vi "Plotter.vi"() -> ()   [LabVIEW 2009]
uses:
  <vilib>/Utility/miscctls.llb/LVPositionTypeDef.ctl
  <vilib>/Utility/tcp.llb/UDP Multicast Read-Only Open.vi
  General-Controler/Stop button.ctl
  <vilib>/Utility/file.llb/Read From Spreadsheet File (string).vi
  <userlib>/_OpenG.lib/array/array.llb/Search 1D Array (String)__ogtk.vi
  <vilib>/Utility/miscctls.llb/LVRectTypeDef.ctl
panel:
  out "Axis Name List":string[](array[string])
  out "Y Axis Default name":string
  out "All Devices Core Info":string[][](array[string])
  out "IP Addresses":string[](array[string])
  out "error out":errorcluster
  out "Position 2":T1
  out "Position":T1
  out "MY IP":string
  out "UDP Mcast Error":errorcluster
  out "Shot #":string
  in  "Tab Control 2":T2(tab)
  out "expt config file array":string[][](array[string])
  out "parameters to get":string[][](array[string])
  out "devices to get data from":string[](array[string])
  out "ScanData to receive":string[][](array[string])
  out "ShotData":string[](array[string])
  out "All shot data":string[][](array[string])
  out "TCP Ports":refnum<k5>[](array[refnum])
  out "Array":errorcluster[](array[cluster])
  in  "Tab Control":enum32{"Main", "ShotData", "setup"}(tab)
  out "xy graph":cluster{dbl[], dbl[]}(graph)={[1.0, 1.0, 1.0, 1.0, 1.0, 1.0, 1.0], [-1.0, -1.0, -1.0, -1.0, -1.0, -1.0, -1.0]}
  in  "Y Axis":u16(ring) items=["Cam1 exposure", "Cam1 trigger", "Cam1 gain", "Cam1Analysis centroidx"]
  in  "X Axis":u16(ring)=1 items=["Cam1 exposure", "Cam1 trigger", "Cam1 gain", "Cam1Analysis centroidx"]
  in  "OK Button":bool
  out "Energy transmission 2":cluster{"y vector":dbl[], "avg optspec":dbl[]}[](graph)
  in  "Fixed Interval":bool
  in  "Interval":dbl format="%.3p"
  in  "Auto Interval":bool
  in  "Error Bar Type":T3(ring)
  in  "Experiment":u16(ring) items=["Cam1only.txt", "Test Startup config.txt", "TREX-Standard.txt"]
  out "Current State":string
  out "Mcast Data":string
  out "Devices Data Timed out":string[](array[string])
  in  "Left":i16=25
  in  "Top":i16=75
  out "x axis name":string
  in  "TCP Open timeout ms":i32=300
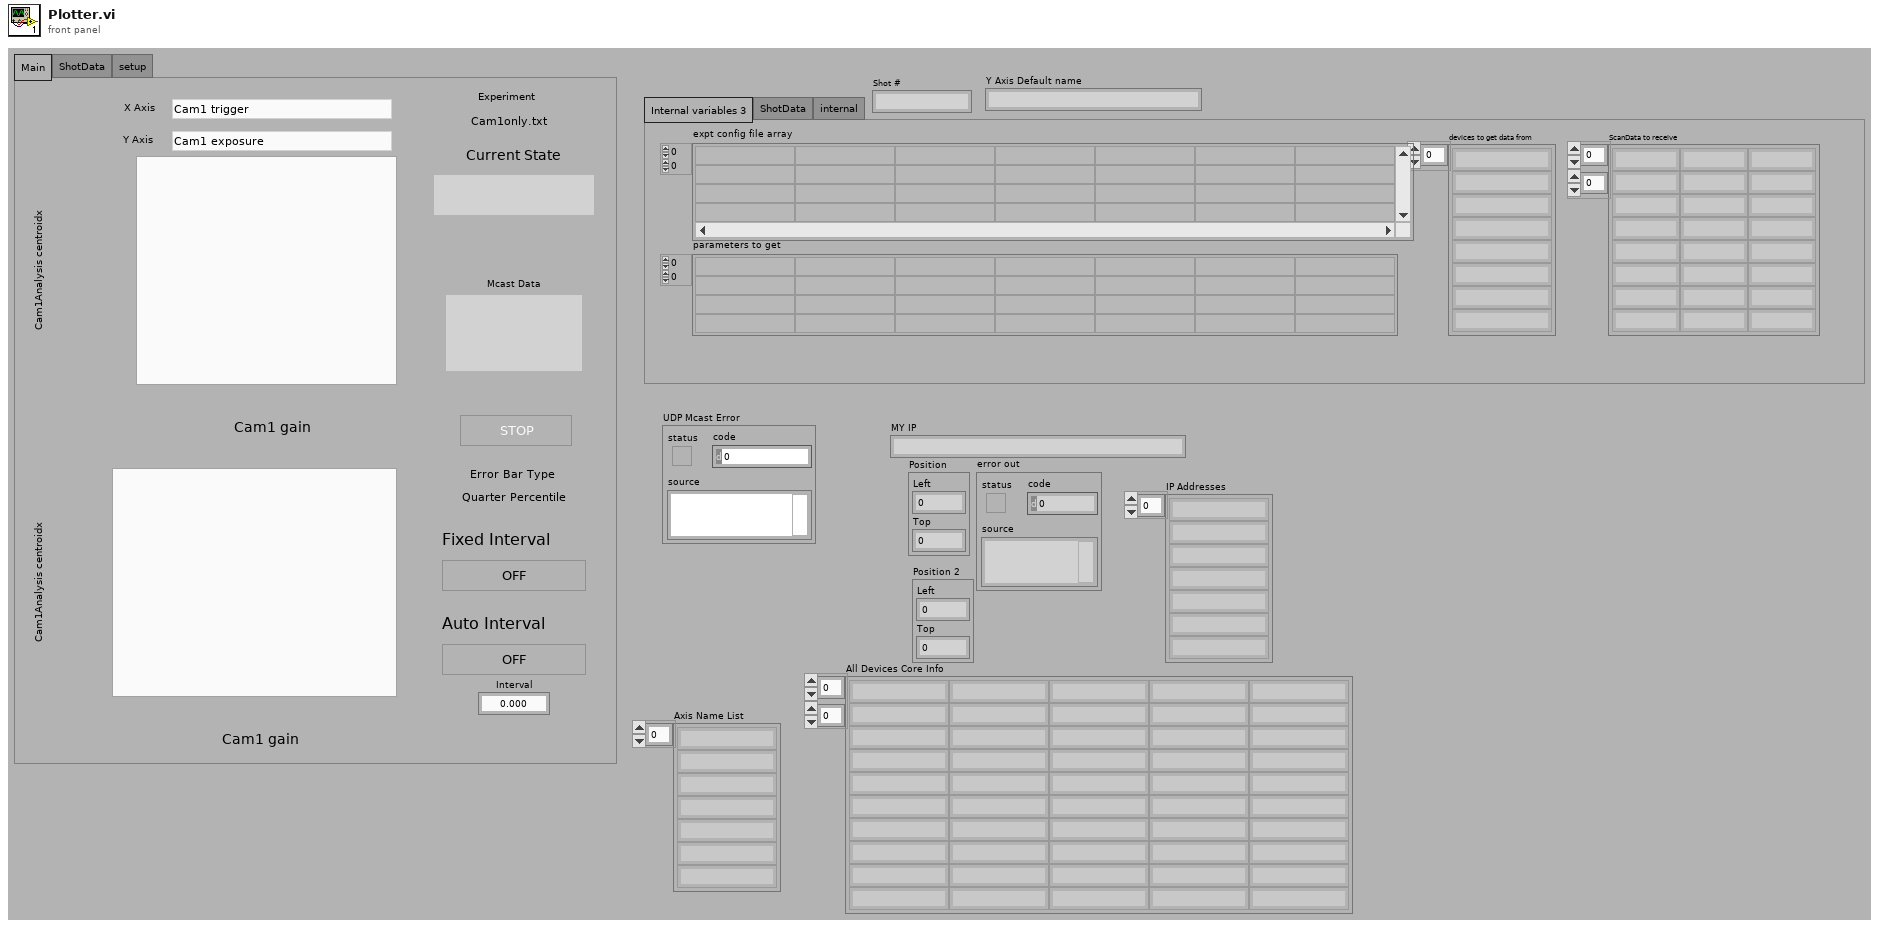
[diagram p1: front panel]
types:
  T1 = typedef "LVPositionTypeDef.ctl" = cluster{"Left":i32, "Top":i32}
  T2 = enum32{"Internal variables 3", "ShotData", "internal"}
  T3 = enum16{"Quarter Percentile", "Standard Deviation"}
  T4 = typedef "Stop button.ctl" = bool
  T5 = enum32{"invalid app kind", "Development System", "Run Time System", "Student Edition", "Embedded LabVIEW", "Evaluation", "Custom"}
  T6 = enum32{"Invalid", "Standard", "Closed", "Hidden", "Minimized", "Maximized"}
  T7 = typedef "LVRectTypeDef.ctl" = cluster{"Left":i16, "Top":i16, "Right":i16, "Bottom":i16}
  T8 = cluster{"Core":cluster{"Current VI Reference":refnum<vi>, "Close Panel on Exit?":bool}, "Variable selector":u16, "variable parameters":string[], "list of variables":string[], "UDP Command to send":string, "Device List":string[], "Config path":path, "Devices Selector":u16, "Device Config file array":string[][], "All Devices Core Info":string[][], "Location Filter":u16, "Filtered Device List":string[], "Class Filter":u16, "Command to Send":string, "Devices Path":path, "UDP ID":refnum<k16>, "parameter vals scanned":dbl[], "List Commands Not Executed":string[], "Expected slow response":string, "MCast Address":string, "MCast Local Port":u16, "MCast Remote Port":u16, "UDP timeout ms":i32, "Scan Number":i32, "Shot Number":i32, "Scan Data Titles":string[], "Scan Data Array":dbl[], "Expt Config Files":string[], "Experiment name":string, "UDP fast port":u16, "name":string, "ScanData to receive":string[][], "UDP Listen Ports":u16[], "Device Names for scan data":string[], "ShotData":string[], "Scans Path":path, "Device xxx Path":path, "numeric?":bool, "Last Slow response":string, "Mcast command":string, "Device Status Array":bool[], "expt config file array":string[][], "Shot Data plotter":string[][], "Data titles from config array":string[]}
  T9 = typedef "LVPointTypeDef.ctl" = cluster{"Horizontal":i16, "Vertical":i16}
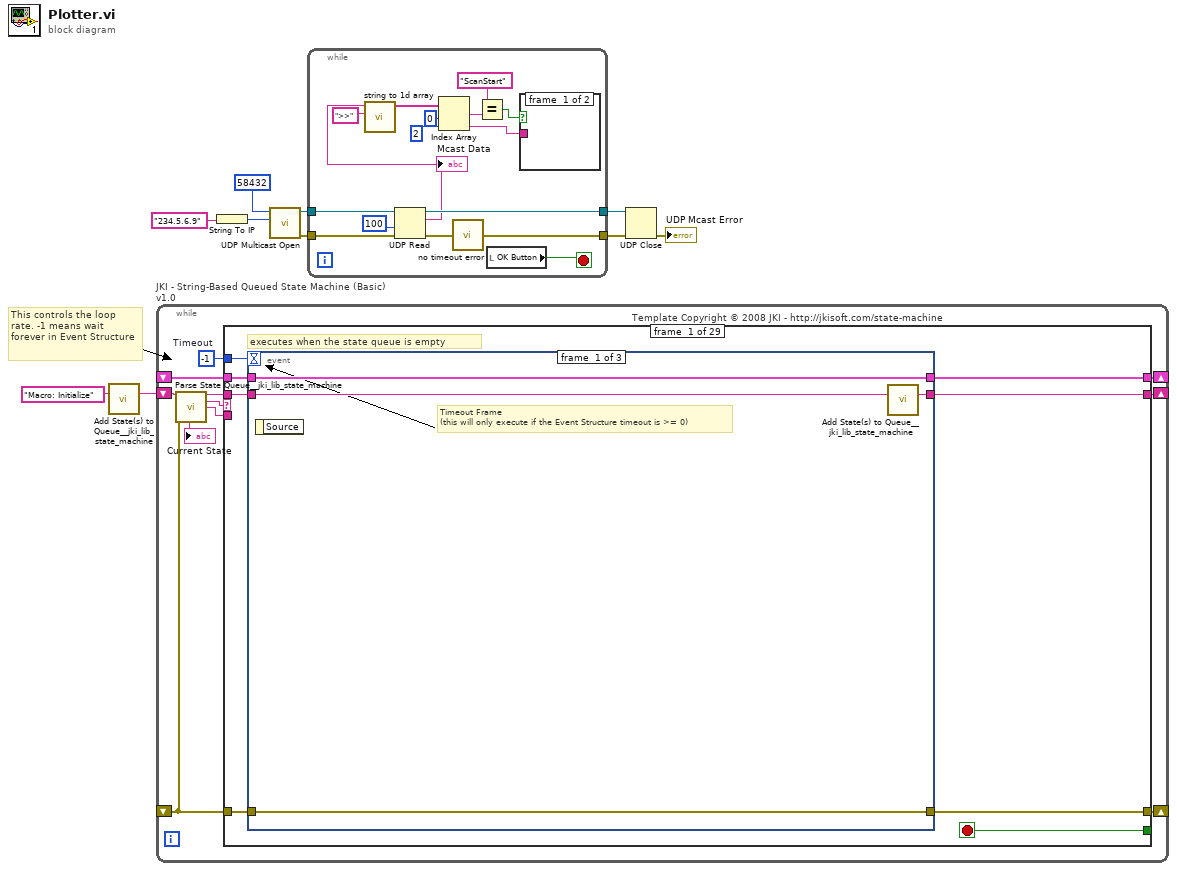
[diagram p0: block diagram]
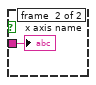
[diagram p2: hidden frame]
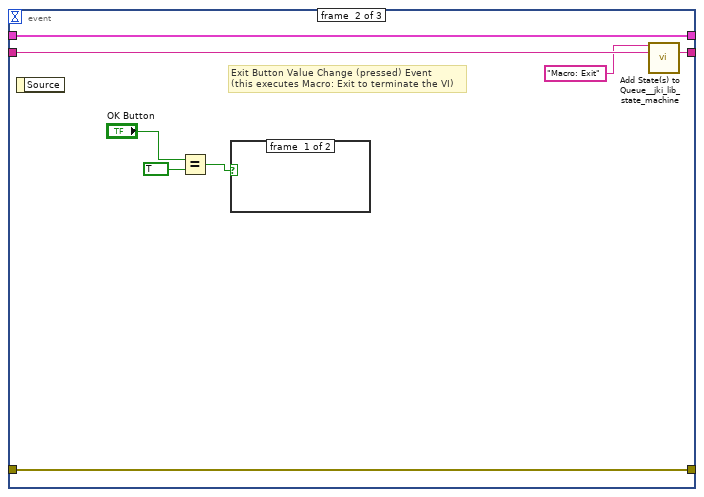
[diagram p3: hidden frame]
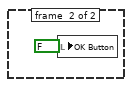
[diagram p4: hidden frame]
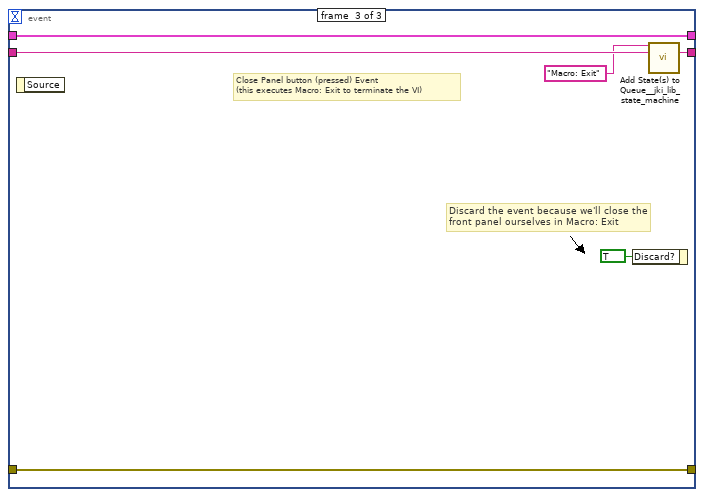
[diagram p5: hidden frame]
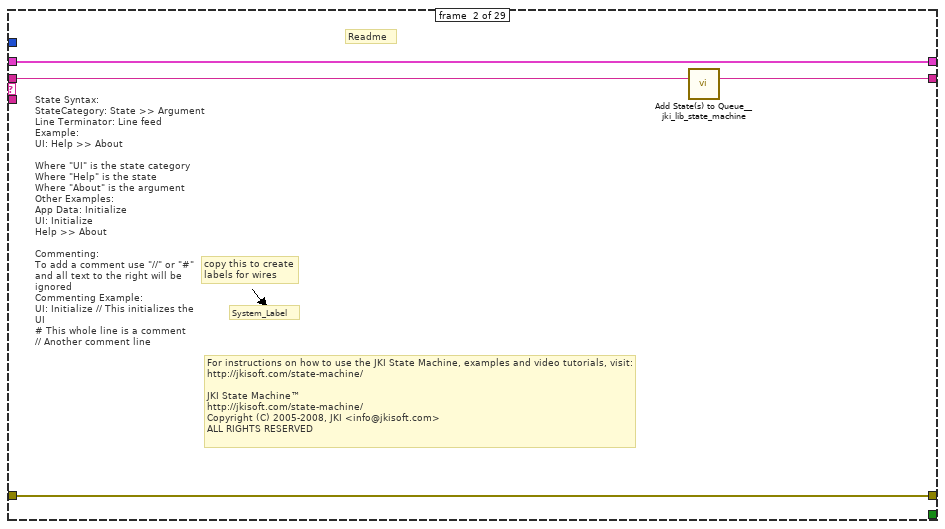
[diagram p6: hidden frame]
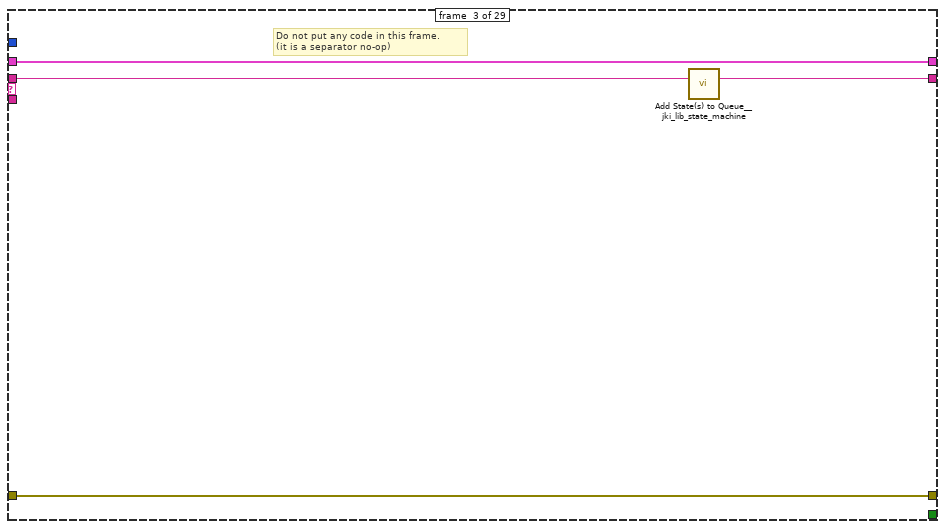
[diagram p7: hidden frame]
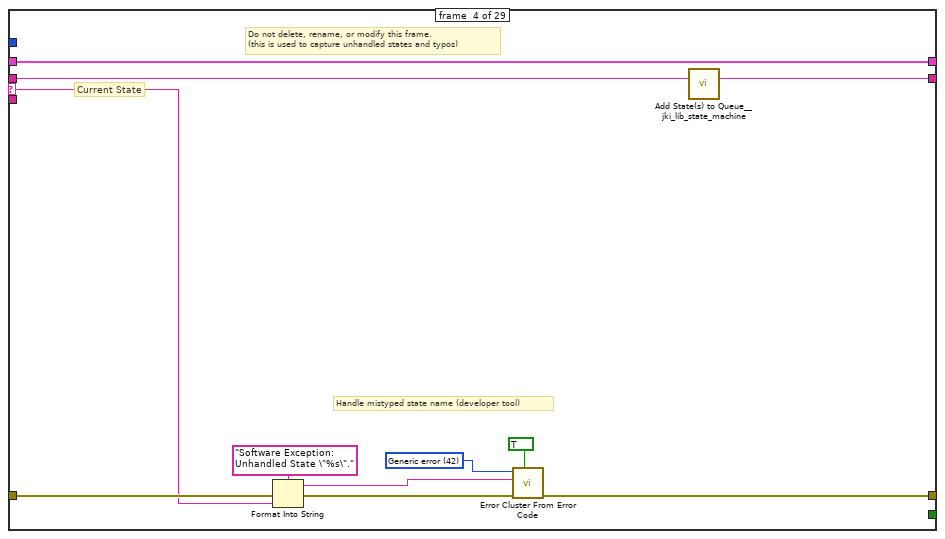
[diagram p8: hidden frame]
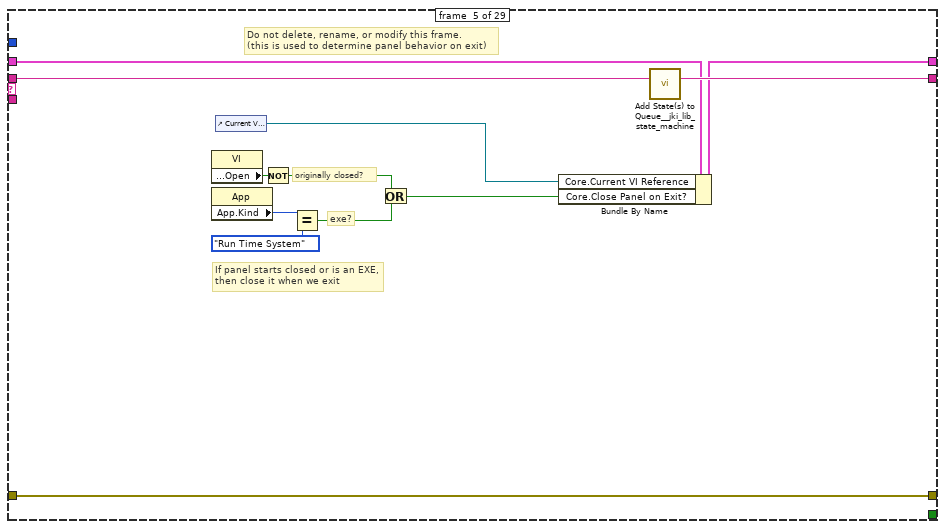
[diagram p9: hidden frame]
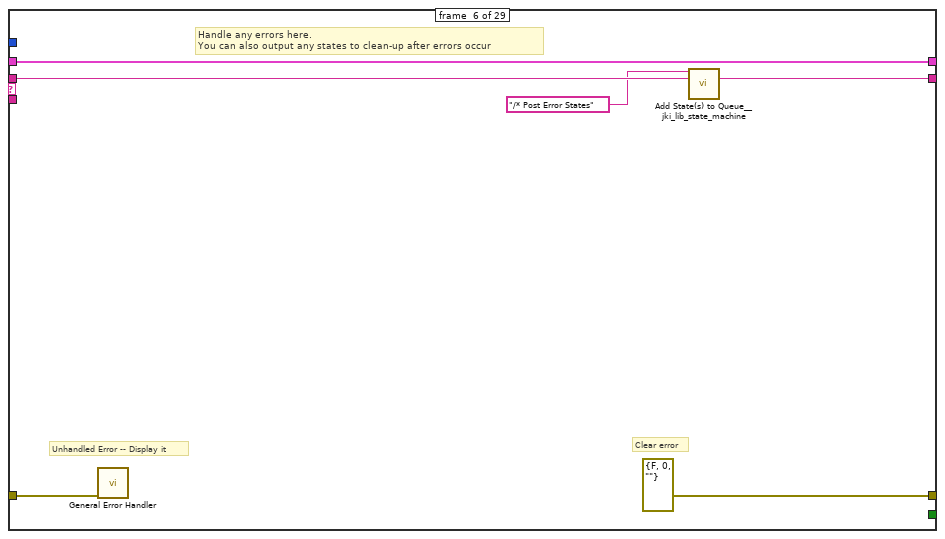
[diagram p10: hidden frame]
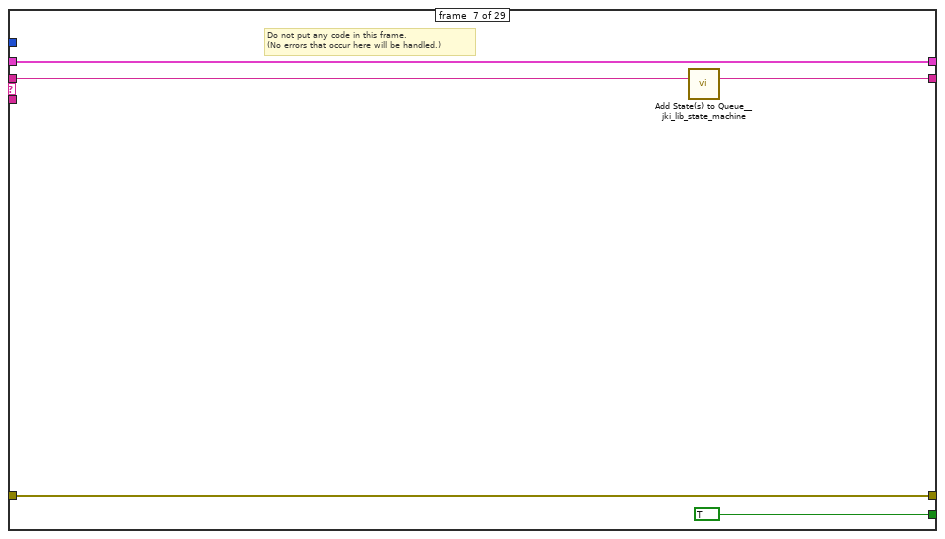
[diagram p11: hidden frame]
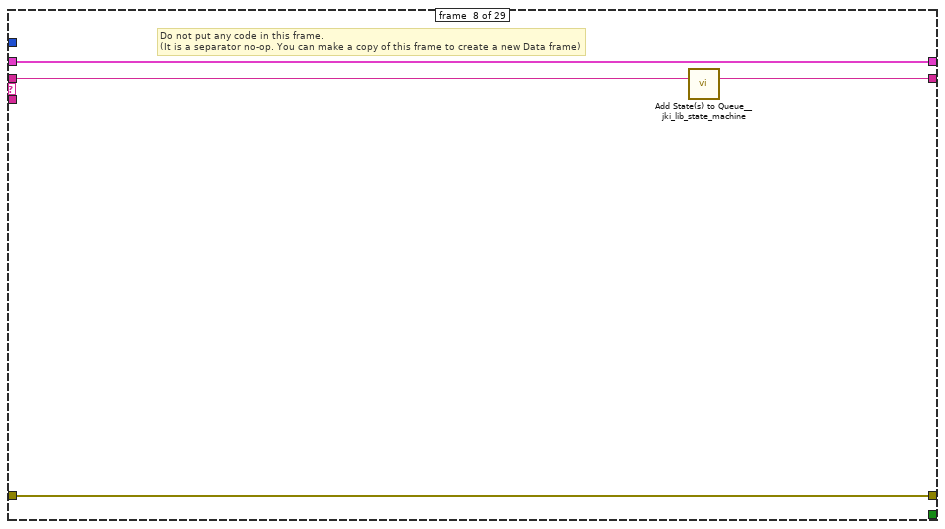
[diagram p12: hidden frame]
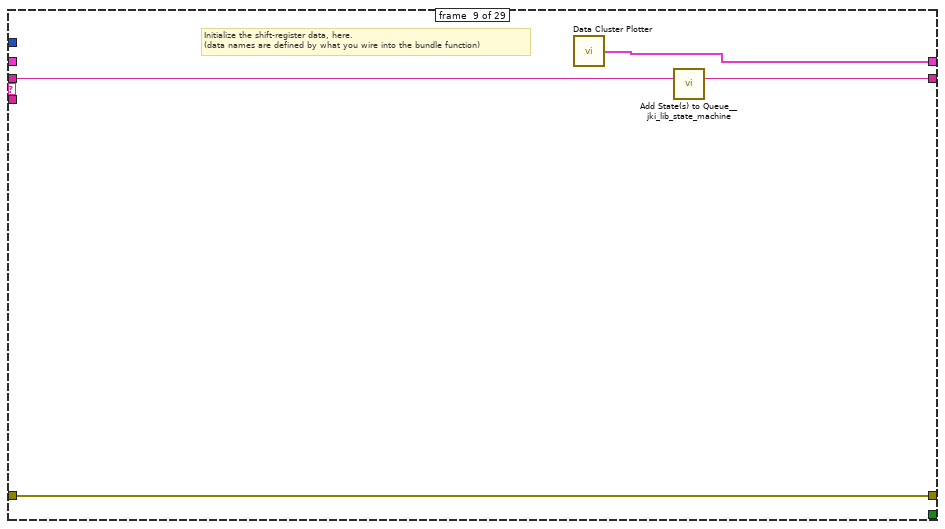
[diagram p13: hidden frame]
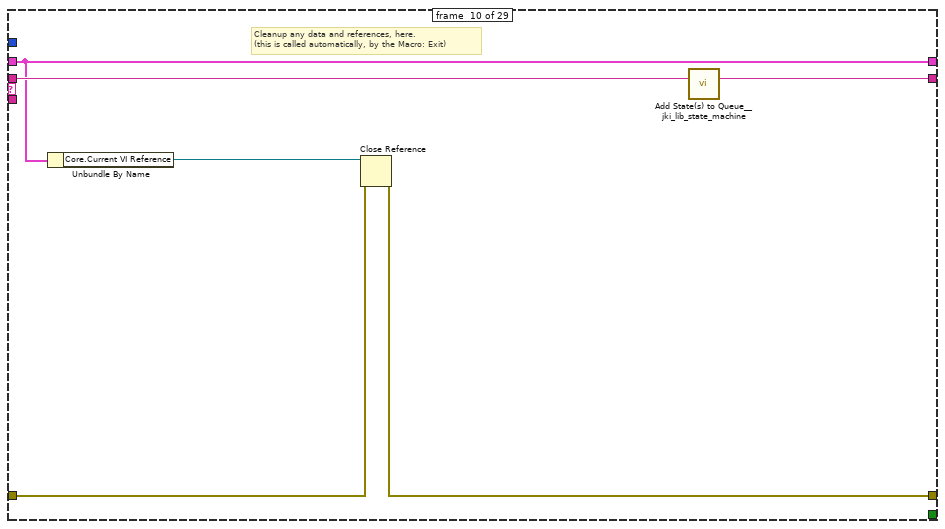
[diagram p14: hidden frame]
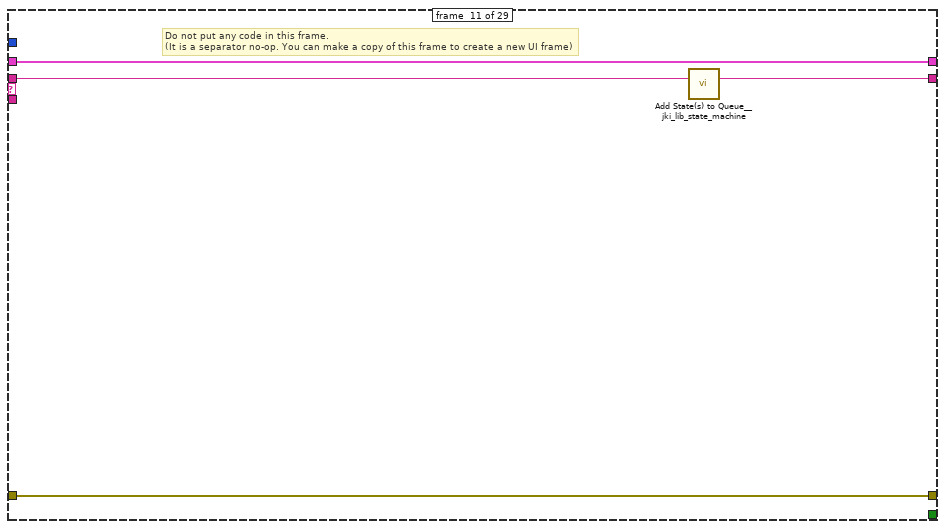
[diagram p15: hidden frame]
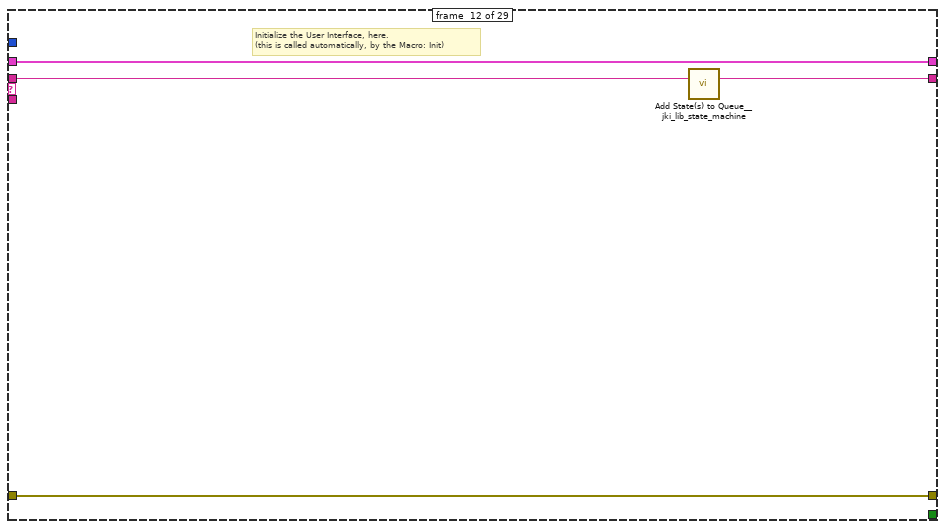
[diagram p16: hidden frame]
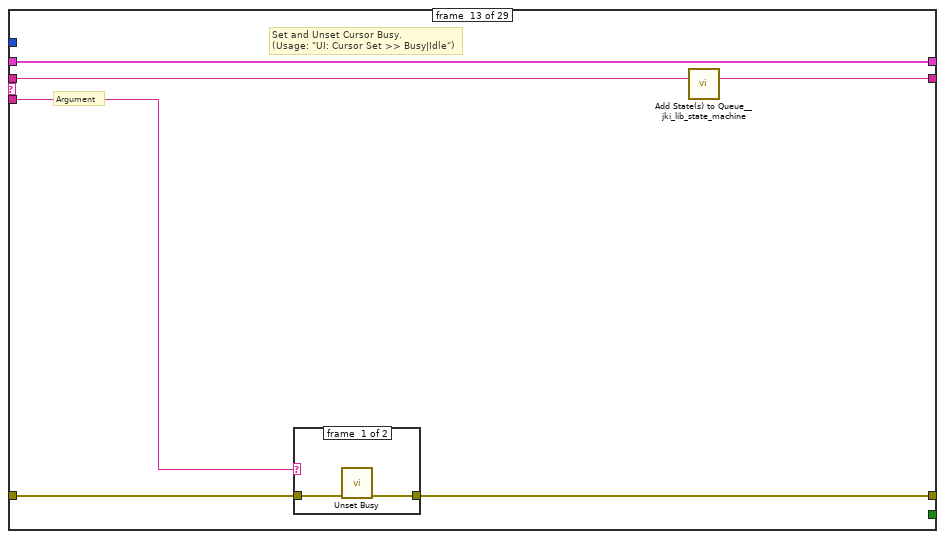
[diagram p17: hidden frame]
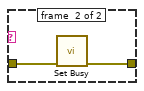
[diagram p18: hidden frame]
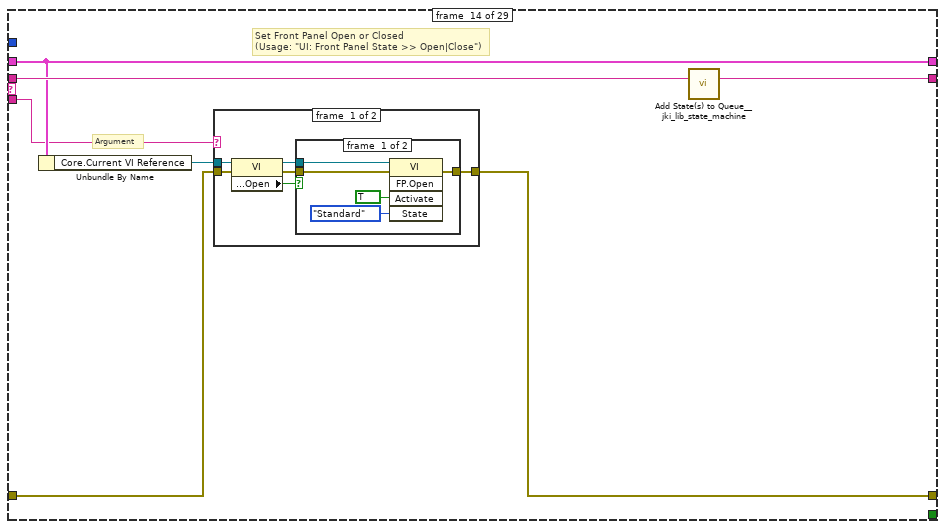
[diagram p19: hidden frame]
diagram:
  # "This controls the loop rate. -1 means wait forever in Event Structure"
  n1 = call <vilib>:"Add State(s) to Queue__jki_lib_state_machine.vi"("State(s) in (\"\")"="Macro: Initialize") -> ("States Out"=w10:string)  [unwired: 14 in]
  n2 = while "JKI - String-Based Queued State Machine (Basic) v1.0" {
    shift-right: [w14] -> _
    shift-left: _ -> [w13]
    shift-right: [w17] -> _
    shift-left: _ -> [w11]
    shift-right: [w16] -> _
    shift-left: w10 -> [w18]
    stop <- w15 stop-if-true
    w12 = -1  # Timeout
    # "Template Copyright © 2008 JKI - http://jkisoft.com/state-machine"
    n3 = call <vilib>:"Parse State Queue__jki_lib_state_machine.vi"("State Queue"=w18, "Error In (no error)"=w11) -> ("Remaining States"=w20:string, "Current State"=w21:string, "Arguments"=w19:string)  [unwired: 11 in]
    "Current State" <- w21
    n4 = case shown="\"Get List of Axis Names\"" w21 {
      selector: w21 -> [_ _ _ w56 _ _ _ _ _ _ _ _ _ _ _ _ _ _ _ _ _ _ _ _ _ _ _ _ _]
      tunnel: w20 -> [w28 w51 w55 w60 w78 w84 w89 w93 w97 w103 w107 w111 w117 w128 w154 w159 w169 w173 w179 w188 w196 w218 w232 w255 w283 w291 w307 w326 w380]
      tunnel: w19 -> [_ _ _ _ _ _ _ _ _ _ _ _ w112 w122 _ _ _ _ _ _ _ _ _ _ _ _ _ _ _]
      tunnel: w13 -> [w26 w48 w52 w58 w69 w81 w87 w90 _ w98 w104 w109 w115 w124 w151 w155 w167 w170 w176 w183 w194 w211 w223 w244 w280 w284 w295 w322 w377]
      tunnel: [w25 w49 w53 w62 w75 errorcluster {"status"=FALSE, "code"=0, "source"=""} ("error out") w86 w91 w95 w99 w105 w108 w113 w125 w152 w157 w160 w171 w177 w180 w191 w199 w230 w253 w281 w289 w293 w324 w378] -> w17
      tunnel: w11 -> [w24 w49 w53 w61 w75 w80 w86 w91 w95 w100 w105 w108 w114 w126 w152 w157 w160 w171 w177 w181 w191 w200 w230 w253 w281 w289 w293 w324 w378]
      tunnel: [w27 w50 w54 w59 w77 w83 w88 w92 w96 w102 w106 w110 w116 w127 w153 w158 w168 w172 w178 w187 w195 w217 w231 w254 w282 w290 w306 w325 w379] -> w16
      tunnel: [_ _ _ _ _ _ TRUE _ _ _ _ _ _ _ _ _ _ _ _ _ _ _ _ _ _ _ _ _ _] -> w15
      tunnel: [w23 w48 w52 w58 w76 w81 w87 w90 w94 w98 w104 w109 w115 w124 w151 w155 w167 w170 w176 w182 w193 w210 w222 w244 w280 w285 w295 w322 w377] -> w14
      tunnel: w12 -> [w22 _ _ _ _ _ _ _ _ _ _ _ _ _ _ _ _ _ _ _ _ _ _ _ _ _ _ _ _]
      frame #0 {
        # "executes when the state queue is empty"
        n5 = event shown="[1] \"OK Button\": Value Change" {
          selector: _ -> [_ _ _]
          dyn-events: _ -> [_ _ _]
          timeout: w22 -> [_ _ _]
          tunnel: w28 -> [w32 w40 w47]
          tunnel: [w31 w39 w46] -> w27
          tunnel: w26 -> [w29 w37 w44]
          tunnel: [w30 w38 w45] -> w25
          tunnel: w24 -> [w30 w38 w45]
          tunnel: [w29 w37 w44] -> w23
          event #0 {
            # "Timeout Frame\n(this will only execute if the Event Structure timeout is >= 0)"
            n6 = event-data() -> ()  [unwired: 1 in, 1 out]
            n7 = call <vilib>:"Add State(s) to Queue__jki_lib_state_machine.vi"("State(s) in (\"\")"=w32) -> ("States Out"=w31:string)  [unwired: 14 in]
          }
          event #1 {
            # "Exit Button Value Change (pressed) Event\n(this executes Macro: Exit to terminate the VI)"
            n8 = event-data() -> ()  [unwired: 1 in, 1 out]
            n9 = Equal?(x="OK Button", y=T4 TRUE) -> (x = y?=w33:T4)
            n10 = case shown="True" w33 {
              frame #0 {
              }
              frame #1 {
                n11 = local write "OK Button"(T4 FALSE ("STOP")) -> ()
              }
            }
            n12 = call <vilib>:"Add State(s) to Queue__jki_lib_state_machine.vi"("State(s) in Front (\"\")"="Macro: Exit", "State(s) in (\"\")"=w40) -> ("States Out"=w39:string)  [unwired: 13 in]
          }
          event #2 {
            # "Discard the event because we'll close the front panel ourselves in Macro: Exit"
            # "Close Panel button (pressed) Event\n(this executes Macro: Exit to terminate the VI)"
            n13 = event-data() -> ()  [unwired: 1 in, 1 out]
            n14 = event-data("Discard?"=TRUE) -> ()  [unwired: 1 in, 1 out]
            n15 = call <vilib>:"Add State(s) to Queue__jki_lib_state_machine.vi"("State(s) in Front (\"\")"="Macro: Exit", "State(s) in (\"\")"=w47) -> ("States Out"=w46:string)  [unwired: 13 in]
          }
        }
      }
      frame #1 {
        # "For instructions on how to use the JKI State Machine, examples and video tutorials, visit:\nhttp://jkisoft.com/state-machine/\n\nJKI State Machine™\nhttp://jkisoft.com/state-machine/\nCopyright (C) 2005-2008, JKI <info@jkisoft.com>\nALL RIGHTS RESERVED"
        # "copy this to create labels for wires"
        # "System_Label"
        # "State Syntax:\nStateCategory: State >> Argument\nLine Terminator: Line feed\nExample:\nUI: Help >> About\n\nWhere \"UI\" is the state category\nWhere \"Help\" is the state\nWhere \"About\" is the argument\nOther Examples:\nApp Data: Initialize\nUI: Initialize\nHelp >> About\n\nCommenting:\nTo add a comment use \"//\" or \"#\" and all text to the right will be ignored\nCommenting Example:\nUI: Initialize // This initializes the UI\n# This whole line is a comment\n// Another comment line"
        # "Readme"
        n16 = call <vilib>:"Add State(s) to Queue__jki_lib_state_machine.vi"("State(s) in (\"\")"=w51) -> ("States Out"=w50:string)  [unwired: 14 in]
      }
      frame #2 {
        # "Do not put any code in this frame.\n(it is a separator no-op)"
        n17 = call <vilib>:"Add State(s) to Queue__jki_lib_state_machine.vi"("State(s) in (\"\")"=w55) -> ("States Out"=w54:string)  [unwired: 14 in]
      }
      frame #3 {
        w65 = 42 items=["No error", "Argument error", "Memory is full", "Out of zone", "End of file", "File already open", "Generic file I/O error", "File not found", "File permission error", "Disk is full", "Duplicate path", "Too many files open", "System feature not enabled", "Resource file not found", "Cannot add resource", "Resource not found", "Image not found", "Image memory error", "Pen does not exist", "Config type invalid", "Config token not found", "Config parse error", "Config memory error", "Bad external code format", "Bad external code offset", "External code not present", "Null window", "Destroy window error", "Null menu", "Print aborted", "Bad print record", "Print driver error", "Windows error during printing", "Memory error during printing", "Print dialog error", "Generic print error", "Invalid device refnum", "Device not found", "Device parameter error", "Device unit error", "Cannot open device", "Device call aborted", "Generic error", "Cancelled by user", "Object ID too low", "Object ID too high", "Object not in heap", "Unknown heap", "Unknown object (invalid DefProc)", "Unknown object (DefProc not in table)", "Message out of range", "Invalid (null) method", "Unknown message", "Manager call not supported", "Bad address", "Network operation in progress", "Network operation timed out", "Connection is busy", "Network attribute not supported", "Network error", "Address in use", "System out of memory", "Connection aborted", "Connection refused", "Not connected", "Already connected", "Connection closed", "Initialization error (interapplication manager)", "Bad occurrence", "Wait on unbound occurrence handler", "Occurrence queue overflow", "Datalog type conflict", "Unused", "Unrecognized type (interapplication manager)", "Memory corrupt", "Failed to make temporary DLL", "Old CIN version", "Drag socket not found", "Failed to load drop-object", "Failed to register OLE object", "Failed to release OLE object", "Format specifier type mismatch", "Unknown format specifier", "Too few format specifiers", "Too many format specifiers", "Scan failed", "Newer CIN version", "Error converting to variant", "Runtime menu error", "Password tampered", "Variant attribute not found", "Incompatible variant data type", "Event data is not available", "Event Store is not present", "Occurrence is not found", "Event Queue is not created", "Event info is not available", "Refnum passed is NULL", "Error retrieving Class GUID", "Error retrieving CoClass GUID", "Error retrieving TypeLib GUID.", "Bad built application magic bytes.", "Specific driver is different from the specific driver associated with the Logical Name.", "There is no session opened to the class driver.", "Max Error", "MAX - Error with config objects", "MAX - Error loading configuration", "MAX - Group not supported"]
        # "Current State"
        # "Do not delete, rename, or modify this frame.\n(this is used to capture unhandled states and typos)"
        # "Handle mistyped state name (developer tool)"
        n18 = Format Into String(format string="Software Exception: Unhandled State \"%s\"." ("message"), error in=w61, w56) -> (resulting string=w64:string, error out=w63:errorcluster)  [unwired: 1 in]
        n19 = call <vilib>:"Error Cluster From Error Code.vi"("show call chain? (False)"=TRUE, "error in (no error)"=w63, "error message (\"\")"=w64, "error code (0)"=w65) -> ("error out"=w62:errorcluster)  [unwired: 5 in]
        n20 = call <vilib>:"Add State(s) to Queue__jki_lib_state_machine.vi"("State(s) in (\"\")"=w60) -> ("States Out"=w59:string)  [unwired: 14 in]
      }
      frame #4 {
        # "Do not delete, rename, or modify this frame.\n(this is used to determine panel behavior on exit)"
        # "originally closed?"
        # "exe?"
        # "If panel starts closed or is an EXE, then close it when we exit"
        n21 = property class="VI"() -> ("Front Panel.Open"=w74:bool)  [unwired: 2 in, 2 out]
        n22 = property class="App"() -> ("App.Kind"=w73:T5)  [unwired: 2 in, 2 out]
        n23 = control-ref of="Current VI Reference"() -> (w67:refnum<vi>)
        n24 = Not(x=w74) -> (.not. x?=w71:bool)
        n25 = Equal?(x=w73, y=T5."Run Time System" ("Application:Kind")) -> (x = y?=w70:bool)
        n26 = Or(x=w71, y=w70) -> (x .or. y?=w68:bool)
        n27 = Bundle By Name(cluster=w69, "Core.Current VI Reference"=w67, "Core.Close Panel on Exit?"=w68) -> (w76:T8)
        n28 = call <vilib>:"Add State(s) to Queue__jki_lib_state_machine.vi"("State(s) in (\"\")"=w78) -> ("States Out"=w77:string)  [unwired: 14 in]
      }
      frame #5 {
        # "Unhandled Error -- Display it"
        # "Handle any errors here.\nYou can also output any states to clean-up after errors occur"
        # "Clear error"
        n29 = call <vilib>:"General Error Handler.vi"("error in (no error)"=w80) -> ()  [unwired: 10 in, 5 out]
        n30 = call <vilib>:"Add State(s) to Queue__jki_lib_state_machine.vi"("State(s) in Front (\"\")"="/* Post Error States", "State(s) in (\"\")"=w84) -> ("States Out"=w83:string)  [unwired: 13 in]
      }
      frame #6 {
        # "Do not put any code in this frame.\n(No errors that occur here will be handled.)"
        n31 = call <vilib>:"Add State(s) to Queue__jki_lib_state_machine.vi"("State(s) in (\"\")"=w89) -> ("States Out"=w88:string)  [unwired: 14 in]
      }
      frame #7 {
        # "Do not put any code in this frame.\n(It is a separator no-op. You can make a copy of this frame to create a new Data frame)"
        n32 = call <vilib>:"Add State(s) to Queue__jki_lib_state_machine.vi"("State(s) in (\"\")"=w93) -> ("States Out"=w92:string)  [unwired: 14 in]
      }
      frame #8 {
        # "Initialize the shift-register data, here.\n(data names are defined by what you wire into the bundle function)"
        n33 = call "Data Cluster Plotter.vi"() -> ("output cluster"=w94:T8)
        n34 = call <vilib>:"Add State(s) to Queue__jki_lib_state_machine.vi"("State(s) in (\"\")"=w97) -> ("States Out"=w96:string)  [unwired: 14 in]
      }
      frame #9 {
        # "Cleanup any data and references, here.\n(this is called automatically, by the Macro: Exit)"
        n35 = Unbundle By Name(w98) -> ("Core.Current VI Reference"=w101:refnum<vi>)
        n36 = Close Reference(reference=w101, error in (no error)=w100) -> (error out=w99:errorcluster)
        n37 = call <vilib>:"Add State(s) to Queue__jki_lib_state_machine.vi"("State(s) in (\"\")"=w103) -> ("States Out"=w102:string)  [unwired: 14 in]
      }
      frame #10 {
        # "Do not put any code in this frame.\n(It is a separator no-op. You can make a copy of this frame to create a new UI frame)"
        n38 = call <vilib>:"Add State(s) to Queue__jki_lib_state_machine.vi"("State(s) in (\"\")"=w107) -> ("States Out"=w106:string)  [unwired: 14 in]
      }
      frame #11 {
        # "Initialize the User Interface, here.\n(this is called automatically, by the Macro: Init)"
        n39 = call <vilib>:"Add State(s) to Queue__jki_lib_state_machine.vi"("State(s) in (\"\")"=w111) -> ("States Out"=w110:string)  [unwired: 14 in]
      }
      frame #12 {
        # "Argument"
        # "Set and Unset Cursor Busy.\n(Usage: \"UI: Cursor Set >> Busy|Idle\")"
        n40 = case shown="\"Idle\", Default" w112 {
          tunnel: w114 -> [w119 w121]
          tunnel: [w118 w120] -> w113
          frame #0 {
            n41 = call <vilib>:"Unset Busy.vi"("error in (no error)"=w119) -> ("error out"=w118:errorcluster)  [unwired: 10 in]
          }
          frame #1 {
            n42 = call <vilib>:"Set Busy.vi"("error in (no error)"=w121) -> ("error out"=w120:errorcluster)  [unwired: 9 in, 1 out]
          }
        }
        n43 = call <vilib>:"Add State(s) to Queue__jki_lib_state_machine.vi"("State(s) in (\"\")"=w117) -> ("States Out"=w116:string)  [unwired: 14 in]
      }
      frame #13 {
        # "Argument"
        # "Set Front Panel Open or Closed\n(Usage: \"UI: Front Panel State >> Open|Close\")"
        n44 = Unbundle By Name(w124) -> ("Core.Current VI Reference"=w123:refnum<vi>)
        n45 = case shown="\"Open\", Default" w122 {
          tunnel: w126 -> [w132 w145]
          tunnel: [w134 w146] -> w125
          tunnel: w123 -> [w133 w143]
          frame #0 {
            n46 = property class="VI"(reference=w133, error in=w132) -> (reference out=w130:refnum<vi>, error out=w131:errorcluster, "Front Panel.Open"=w129:bool)
            n47 = case shown="True" w129 {
              tunnel: [w137 w140] -> w134
              tunnel: w131 -> [w136 w140]
              tunnel: w130 -> [w135 _]
              frame #0 {
                n48 = invoke class="VI" method="FP.Open"(reference=w135, error in=w136, "Activate"=TRUE, "State"=T6."Standard") -> (error out=w137:errorcluster)  [unwired: 1 in, 4 out]
              }
              frame #1 {
              }
            }
          }
          frame #1 {
            n49 = property class="VI"(reference=w143, error in=w145) -> (reference out=w142:refnum<vi>, error out=w144:errorcluster, "Front Panel.Open"=w141:bool)
            n50 = case shown="True" w141 {
              tunnel: [w147 w150] -> w146
              tunnel: w144 -> [w147 w149]
              tunnel: w142 -> [_ w148]
              frame #0 {
              }
              frame #1 {
                n51 = invoke class="VI" method="FP.Close"(reference=w148, error in=w149) -> (error out=w150:errorcluster)  [unwired: 1 in, 2 out]
              }
            }
          }
        }
        n52 = call <vilib>:"Add State(s) to Queue__jki_lib_state_machine.vi"("State(s) in (\"\")"=w128) -> ("States Out"=w127:string)  [unwired: 14 in]
      }
      frame #14 {
        # "Do not put any code in this frame.\n(It is a separator no-op. You can make a copy of this frame to create a new Macro frame)"
        n53 = call <vilib>:"Add State(s) to Queue__jki_lib_state_machine.vi"("State(s) in (\"\")"=w154) -> ("States Out"=w153:string)  [unwired: 14 in]
      }
      frame #15 {
        w156 = "Data: Initialize\nInitialize Core Data\nUI: Initialize\nUI: Front Panel State >> Open\nMain: Macro"  # Data: Initialize Initialize Core Data UI: Initialize UI: Front Panel State >> Open Main: Macro
        # "Initialization Macro\n(This is called once, when the VI starts)"
        n54 = call <vilib>:"Add State(s) to Queue__jki_lib_state_machine.vi"("State(s) in Front (\"\")"=w156, "State(s) in (\"\")"=w159) -> ("States Out"=w158:string)  [unwired: 13 in]
      }
      frame #16 {
        # "Exit Macro\n(This is called once, when the VI exits)"
        n55 = Unbundle By Name(w167) -> ("Core.Close Panel on Exit?"=w166:bool)
        n56 = Select(t="UI: Front Panel State >> Close", s=w166, f="") -> (s? t:f=w163:string)
        n57 = call <vilib>:"Add State(s) to Queue__jki_lib_state_machine.vi"("State(s) in (\"\")"=w163, "State(s) at Back (\"\")"="Data: Cleanup\nExit") -> ("States Out"=w161:string)  [unwired: 13 in]
        n58 = call <vilib>:"Add State(s) to Queue__jki_lib_state_machine.vi"("State(s) in Front (\"\")"=w161, "State(s) in (\"\")"=w169) -> ("States Out"=w168:string)  [unwired: 13 in]
      }
      frame #17 {
        # "Template Separator\n(You can make a copy of, or modify, this frame)"
        n59 = call <vilib>:"Add State(s) to Queue__jki_lib_state_machine.vi"("State(s) in (\"\")"=w173) -> ("States Out"=w172:string)  [unwired: 14 in]
      }
      frame #18 {
        # "Sets the list of states to execute on vi startup in the first string and  the list of states to execute on each loop\nin the second string"
        n60 = local write "Tab Control"(0) -> ()
        n61 = call <vilib>:"Add State(s) to Queue__jki_lib_state_machine.vi"("State(s) in Front (\"\")"="Main: Read Expt Configs\nMain: Get Expt name\nMain: Read Expt Config\nGet List of Axis Names\nGet Default Y Axis\nMain: Set Panel Postion\nMain: Get Device Configs\nMain: Get Listen Ports\nMain: Get Shot info", "State(s) in (\"\")"=w179) -> ("States Out"=w178:string)  [unwired: 13 in]
      }
      frame #19 {
        # "Gets experimental configuration filenames. These files contain information specific to an experiment. Eg TREX expt\nfile would have all the devices that need to startup and their default variable values."
        n62 = Unbundle By Name(w183) -> ("Devices Path"=w186:path)
        n63 = call "get expt config filenames.vi"("Devices Path"=w186, "error in"=w181) -> ("Expt Config filenames"=w184:string[], "error out"=w180:errorcluster)  [unwired: 1 out]
        n64 = call "array to strings and values for ring.vi"("list of variables"=w184) -> ("Array"=w185:cluster{"String":string, i32}[])
        n65 = property on="Experiment" class="Ring (strict)"("StringsAndValues[]"=w185) -> ()  [unwired: 2 in, 2 out]
        n66 = Bundle By Name(cluster=w183, "Expt Config Files"=w184) -> (w182:T8)
        n67 = call <vilib>:"Add State(s) to Queue__jki_lib_state_machine.vi"("State(s) in (\"\")"=w188) -> ("States Out"=w187:string)  [unwired: 14 in]
      }
      frame #20 {
        # "Increments scan #, resets shot number and sends list of states to execute at the start of a scan. Only does this\nif variable for scan is numeric."
        n68 = Unbundle By Name(w194) -> ("Expt Config Files"=w192:string[])
        n69 = Index Array(array=w192, index="Experiment") -> (element=w190:string)
        n70 = Bundle By Name(cluster=w194, "Experiment name"=w190) -> (w193:T8)
        n71 = call <vilib>:"Add State(s) to Queue__jki_lib_state_machine.vi"("State(s) in (\"\")"=w196) -> ("States Out"=w195:string)  [unwired: 14 in]
      }
      frame #21 {
        # "Reads the configuration for a particular experiment. eg TREX default would save spectrum mode image and\nget back centroid etc."
        n72 = Unbundle By Name(w211) -> ("Devices Path"=w216:path, "Experiment name"=w214:string)
        n73 = call "get expt config filenames.vi"("Devices Path"=w216, "error in"=w200) -> ("Expt Config Folder"=w215:path, "error out"=w201:errorcluster)  [unwired: 1 out]
        n74 = Build Path(base path=w215, name or relative path=w214) -> (appended path=w203:path)
        n75 = call <vilib>:"Check if File or Folder Exists.vi"("error in (no error)"=w201, "path"=w203) -> ("error out"=w199:errorcluster, "file or folder exists?"=w198:bool, "dup path"=w202:path)  [unwired: 7 in]
        n76 = case shown="True" w198 {
          tunnel: [_ w220] -> w197
          tunnel: w202 -> [_ w219]
          frame #0 {
          }
          frame #1 {
            n77 = call-poly <vilib>:"Read From Spreadsheet File.vi"("format (%s)"="%s" ("format (%.3f)"), "file path (dialog if empty)"=w219) -> ("all rows"=w220:string[][])  [unwired: 5 in, 4 out]
          }
        }
        "expt config file array" <- w197
        n78 = call "filter array based upon column value.vi"("Reject if Column is ="="no" ("Element Data"), "Input Array"=w197, "Column Title"="get") -> ("array only w/ rejected columns"=w209:string[][])  [unwired: 1 out]
        n79 = Delete From Array(array=w209, length=3, index (col)=2 ("disabled index (col)")) -> (array with subset deleted=w205:string[][])  [unwired: 1 in, 1 out]
        "parameters to get" <- w205
        n80 = call "remove rows of duplicate col in 2d array.vi"("column to find dups"=0, "2D array"=w205) -> ("unique column values"=w204:string[])  [unwired: 1 out]
        "devices to get data from" <- w204
        n81 = Bundle By Name(cluster=w211, "expt config file array"=w197, "ScanData to receive"=w205, "Device Names for scan data"=w204) -> (w210:T8)
        n82 = call <vilib>:"Add State(s) to Queue__jki_lib_state_machine.vi"("State(s) in (\"\")"=w218) -> ("States Out"=w217:string)  [unwired: 14 in]
      }
      frame #22 {
        # "Increments scan #, resets shot number and sends list of states to execute at the start of a scan. Only does this\nif variable for scan is numeric."
        n83 = Unbundle By Name(w223) -> ("ScanData to receive"=w229:string[][])
        n84 = Index Array(array=w229, index (col) #1=0 ("disabled index (col)"), index (col) #2=1 ("index (col)")) -> (element #1=w226:string[], element #2=w225:string[])  [unwired: 2 in]
        n85 = for {
          tunnel: w226 -> [w235] mode=indexing
          tunnel: w225 -> [w234] mode=indexing
          tunnel: [w233] -> w224 mode=indexing
          n86 = Concatenate Strings(w235, " " ("string"), w234) -> (w233:string)
        }
        "Axis Name List" <- w224
        n87 = property on="X Axis" class="Ring (strict)"("Strings []"=w224) -> ()  [unwired: 2 in, 2 out]
        n88 = property on="Y Axis" class="Ring (strict)"("Strings []"=w224) -> ()  [unwired: 2 in, 2 out]
        n89 = Bundle By Name(cluster=w223, "Data titles from config array"=w224) -> (w222:T8)
        n90 = call <vilib>:"Add State(s) to Queue__jki_lib_state_machine.vi"("State(s) in (\"\")"=w232) -> ("States Out"=w231:string)  [unwired: 14 in]
      }
      frame #23 {
        # "Increments scan #, resets shot number and sends list of states to execute at the start of a scan. Only does this\nif variable for scan is numeric."
        n91 = Unbundle By Name(w244) -> ("expt config file array"=w246:string[][])
        n92 = String To IP() -> (0:w249:u32)  [unwired: 1 in]
        n93 = IP To String(1:TRUE ("dot notation? (F)"), 2:w249) -> (0:w248:string)
        "MY IP" <- w248
        n94 = Index Array(array=w246, index (col)=8 ("disabled index (col)")) -> (element=w251:string[])  [unwired: 1 in]
        n95 = call-poly <userlib>:"Search Array__ogtk.vi"("Array"=w251, "Element Data"=w248) -> ("Indices of Elements"=w247:i32[])  [unwired: 7 in]
        n96 = Index Array(array=w247) -> (element=w245:i32)  [unwired: 1 in]
        n97 = Index Array(array=w246, index (row)=w245) -> (element=w243:string[])  [unwired: 1 in]
        n98 = Index Array(array=w243) -> (element #1=w242:string, element #2=w240:string)  [unwired: 2 in]
        n99 = Concatenate Strings(w242, " " ("string"), w240) -> (w238:string)
        "Y Axis Default name" <- w238
        n100 = property on="Y Axis" class="Ring (strict)"() -> ("Strings []"=w239:string[])  [unwired: 2 in, 2 out]
        n101 = call <vilib>:"Add State(s) to Queue__jki_lib_state_machine.vi"("State(s) in (\"\")"=w255) -> ("States Out"=w254:string)  [unwired: 14 in]
        n102 = Search 1D Array(1D array=w239, element=w238) -> (index of element=w237:i32)  [unwired: 1 in]
        n103 = local write "Y Axis"(w237) -> ()
      }
      frame #24 {
        # "Reads the configuration for a particular experiment. eg TREX default would save spectrum mode image and\nget back centroid etc."
        n104 = control-ref of="This VI"() -> (w272:refnum<vi>)
        n105 = property class="VI"(reference=w272) -> (reference out=w267:refnum<vi>, error out=w265:errorcluster, "Panel"=w274:refnum<vi>)  [unwired: 1 in]
        n106 = property on="Tab Control" class="TabCtl (strict)"() -> ("PaneWidth"=w261:u32, "PaneHeight"=w260:u32)  [unwired: 2 in, 2 out]
        n107 = Add(x=w260, y=u32 25) -> (x+y=w258:u32)
        n108 = Add(x=u32 2, y=w261) -> (x+y=w259:u32)
        n109 = property class="Pnl"(reference=w274, error in=w265) -> (reference out=w268:refnum<vi>, error out=w264:errorcluster, "Position"=→"Position":T1, "Panes[]"=w271:refnum<vi>[])
        n110 = Index Array(array=w271) -> (element=w270:refnum<vi>)  [unwired: 1 in]
        n111 = property class="Pane"(reference=w270, error in=w264) -> (error out=w263:errorcluster, "Origin"=w269:T9)  [unwired: 1 out]
        "Position 2" <- w269
        n112 = Add(x="Top", y=w258) -> (x+y=w279:u32)
        n113 = Add(x="Left", y=w259) -> (x+y=w276:u32)
        n114 = property class="Pnl"(reference=w268, error in=w263, "Position"=w269) -> (error out=w262:errorcluster)  [unwired: 1 out]
        n115 = Bundle By Name(cluster=T7 {"Left"=0, "Top"=0, "Right"=0, "Bottom"=0} ("Front Panel Window:Panel Bounds"), "Left"="Left", "Top"="Top", "Right"=w276, "Bottom"=w279) -> (w266:T7)
        n116 = property class="VI"(reference=w267, error in=w262, "Front Panel.PanelBounds"=w266) -> ()  [unwired: 2 out]
        n117 = call <vilib>:"Add State(s) to Queue__jki_lib_state_machine.vi"("State(s) in (\"\")"=w283) -> ("States Out"=w282:string)  [unwired: 14 in]
      }
      frame #25 {
        # "Reads the configuration for a particular experiment. eg TREX default would save spectrum mode image and\nget back centroid etc."
        n118 = Unbundle By Name(w284) -> ("Devices Path"=w287:path, "Device Names for scan data"=w288:string[])
        n119 = call "get classes and locations.vi"("Device List"=w288, "Path"=w287) -> ("All Devices Core Info"=w286:string[][])
        "All Devices Core Info" <- w286
        n120 = Bundle By Name(cluster=w284, "All Devices Core Info"=w286) -> (w285:T8)
        n121 = call <vilib>:"Add State(s) to Queue__jki_lib_state_machine.vi"("State(s) in (\"\")"=w291) -> ("States Out"=w290:string)  [unwired: 14 in]
      }
      frame #26 {
        # "Here the program gets the UDP ports of devices and anlaysis vis. For things like pressures, centroids. etc. For these devices\nthe vi will wait until the full dataset has been received (but with timeout). Will alert to failed devices."
        n122 = Unbundle By Name(w295) -> ("Device Names for scan data"=w298:string[], "ScanData to receive"=→"ScanData to receive":string[][], "All Devices Core Info"=w304:string[][], "expt config file array"=w299:string[][])
        n123 = for {
          tunnel: w299 -> [w319]
          tunnel: w298 -> [w318] mode=indexing
          tunnel: [w317] -> w297 mode=indexing
          n124 = call "Subscriber read from exp config file array.vi"("whatamI"=w318, "expt config file array"=w319) -> ("Subscribe command"=w317:string)  [unwired: 5 in]
        }
        n125 = call "get info from core device data.vi"("devices to get data from"=w298, "All Devices Core Info"=w304) -> ("Ports"=w302:string[], "IP Addresses"=w303:string[])  [unwired: 2 in]
        "IP Addresses" <- w303
        n126 = while {
          tunnel: w303 -> [w316]
          tunnel: w302 -> [w315]
          tunnel: [w314] -> w301
          tunnel: [w311] -> w296
          tunnel: "TCP Open timeout ms" -> [w308]
          stop <- w313 stop-if-true
          n127 = local read "OK Button"() -> (w312:bool)
          n128 = call "TCP multiple open.vi"("timeout ms (60000)"=w308, "Ports"=w315, "IP Addresses"=w316) -> ("error out"=w311:errorcluster, "Array"=w314:refnum<k5>[])  [unwired: 1 in]
          n129 = Unbundle By Name(w311) -> ("status"=w310:bool)
          n130 = Not(x=w310) -> (.not. x?=w309:bool)
          n131 = Or(x=w309, y=w312) -> (x .or. y?=w313:bool)
        }
        "TCP Ports" <- w301
        n132 = call "tcp multiple write.vi"("Connection ID array"=w301, "error in 1 (no error)"=w296, "messages to send"=w297, "timeout ms (25000)"=300) -> ("error out"=→"error out":errorcluster)
        n133 = call <vilib>:"Add State(s) to Queue__jki_lib_state_machine.vi"("State(s) in (\"\")"=w307) -> ("States Out"=w306:string)  [unwired: 14 in]
      }
      frame #27 {
        # "Here the program gets info from devices and anlaysis vis. eg pressures, centroids. etc. For these devices\nthe vi will wait until the full dataset has been received (but with timeout). Will alert to failed devices."
        n134 = Unbundle By Name(w322) -> ("Data titles from config array"=w320:string[], "Device Names for scan data"=w321:string[])
        n135 = while {
          tunnel: w321 -> [w345]
          shift-right: [w339] -> _
          shift-left: string[][] [] ("ShotData 2") -> [w335]
          tunnel: w320 -> [w330]
          stop <- w340 stop-if-true
          n136 = local read "TCP Ports"() -> (w341:refnum<k5>[])
          n137 = call "tcp multiple read.vi"("timeout ms (25000)"=1000, "TCP Ports"=w341) -> ("Read Errors"=w344:errorcluster[], "Data read by TCP"=w334:string[])
          "ShotData" <- w334
          "Array" <- w344
          n138 = call "get devices with udp no response.vi"("Array 2"=w344, "Device Names for scan data"=w345) -> ("with error"=→"Devices Data Timed out":string[])  [unwired: 1 out]
          n139 = call "Plotter parse device data.vi"("ShotData"=w334) -> ("Shot #"=w333:string)  [unwired: 9 in, 1 out]
          "Shot #" <- w333
          n140 = Equal?(x="1", y=w333) -> (x = y?=w338:bool)
          n141 = Select(t=string[][] [] ("ShotData 2"), s=w338, f=w335) -> (s? t:f=w332:string[][])
          n142 = call "Add to shot data 2d array.vi"("TCP Raw ShotData"=w334, "ShotData 2D array in"=w332, "Array titles from config file"=w330) -> ("ShotData 2D array out"=w331:string[][])  [unwired: 5 in, 3 out]
          n143 = stacked-sequence {
            tunnel: w331 -> [w346 _ _ _ _]
            tunnel: [w346 _ _ _ _] -> w339
            frame #0 {
              n144 = control-ref of="XY Graph"() -> (w350:refnum<vi>)
              n145 = control-ref of="X Axis"() -> (w349:refnum<vi>)
              n146 = control-ref of="Y Axis"() -> (w348:refnum<vi>)
              n147 = call "Select axes.vi"("XYGraph Refnum"=w350, "Ring Refnum"=w349, "Ring Refnum 2"=w348, "output array"=w346) -> ("Cluster"=→"xy graph":cluster{dbl[], dbl[]})  [unwired: 4 out]
              "All shot data" <- w346
            }
            frame #1 {
              n148 = local read "x axis name"() -> (w351:string)
              n149 = property on="X Axis" class="Ring (strict)"() -> ("Strings []"=w353:string[])  [unwired: 2 in, 2 out]
              n150 = Search 1D Array(1D array=w353, element=w351) -> (index of element=w352:i32)  [unwired: 1 in]
              n151 = local write "X Axis"(w352) -> ()
            }
            frame #2 {
              n152 = case shown="True" "Auto Interval" {
                frame #0 {
                }
                frame #1 {
                  n153 = local read "xy graph"() -> (w356:cluster{dbl[], dbl[]})
                  n154 = Unbundle(w356) -> (w355:dbl[])  [unwired: 1 out]
                  n155 = Array Max & Min(array=w355) -> (max value=w358:dbl, min value=w359:dbl)  [unwired: 2 out]
                  n156 = Subtract(x=w358, y=w359) -> (x-y=w360:dbl)
                  n157 = Divide(x=w360, y=10.0) -> (x/y=w357:dbl)
                  n158 = local write "Interval"(w357) -> ()
                }
              }
            }
            frame #3 {
              n159 = property on="xy graph" class="XYGraph (strict)"() -> ("XScale.NameLbl.Text"=w363:string, "YScale.NameLbl.Text"=w362:string)  [unwired: 2 in, 2 out]
              n160 = property on="Energy transmission 2" class="XYGraph (strict)"("XScale.NameLbl.Text"=w363, "YScale.NameLbl.Text"=w362) -> ()  [unwired: 2 in, 2 out]
            }
            frame #4 {
              n161 = local read "xy graph"() -> (w370:cluster{dbl[], dbl[]})
              n162 = Unbundle(w370) -> (w368:dbl[])  [unwired: 1 out]
              n163 = Array Size(array=w368) -> (size(s)=w369:i32)
              n164 = Build Array(w370) -> (w371:cluster{dbl[], dbl[]}[])
              n165 = Not Equal To 0?(x=w369) -> (x != 0?=w366:bool)
              n166 = Not Equal To 0?(x="Interval") -> (x != 0?=w365:bool)
              n167 = And(x=w366, y=w365) -> (x .and. y?=w364:bool)
              n168 = case shown="True" w364 {
                tunnel: w371 -> [_ w376]
                tunnel: "Interval" -> [_ w372]
                frame #0 {
                }
                frame #1 {
                  n169 = call "bin multiple xy graphs-b.vi"("Error Bar Type"="Error Bar Type", "interval"=w372, "FIXED X INTERVAL?"="Fixed Interval", "parameter 2,3,4 vs 1"=w376) -> ("Array"=→"Energy transmission 2":cluster{"y vector":dbl[], "avg optspec":dbl[]}[])  [unwired: 1 out]
                }
              }
            }
          }
          n170 = local read "OK Button"() -> (w340:bool)
        }
        n171 = while {
          stop <- w328 stop-if-true
          n172 = Wait (ms)(milliseconds to wait=u32 200) -> ()  [unwired: 1 out]
          n173 = local read "OK Button"() -> (w328:bool)
          n174 = case shown="True" w328 {
            frame #0 {
            }
            frame #1 {
              n175 = local read "TCP Ports"() -> (w329:refnum<k5>[])
              n176 = call "TCP multi close.vi"("TCP Ports"=w329) -> ()
            }
          }
        }
        n177 = call <vilib>:"Add State(s) to Queue__jki_lib_state_machine.vi"("State(s) in (\"\")"=w326) -> ("States Out"=w325:string)  [unwired: 14 in]
      }
      frame #28 {
        # "Your code here.\n(You can make a copy of, or modify, this frame)"
        n178 = call <vilib>:"Add State(s) to Queue__jki_lib_state_machine.vi"("State(s) in (\"\")"=w380) -> ("States Out"=w379:string)  [unwired: 14 in]
      }
    }
  }
  n179 = String To IP(1:"234.5.6.9" ("Multicast Address")) -> (0:w7:u32)
  n180 = call-poly <vilib>:"UDP Multicast Open.vi"("multicast addr"=w7, "port"=58432 ("Port")) -> ("error out"=w1:errorcluster, "connection ID"=w5:refnum<k16>)  [unwired: 7 in, 1 out]
  n181 = while {
    tunnel: w5 -> [w395]
    tunnel: [w392] -> w4
    tunnel: [w391] -> w3
    tunnel: w1 -> [w381]
    stop <- w393 stop-if-true
    n182 = UDP Read(connection ID=w395, timeout ms (25000)=100, 8:w381) -> (data out=w383:string, error out=w394:errorcluster, 3:w392:refnum<k16>)  [unwired: 3 out]
    "Mcast Data" <- w383
    n183 = call "string to 1d array.vi"("delimiter (Tab)"=">>", "string"=w383) -> ("Array of Strings"=w388:string[])  [unwired: 9 in]
    n184 = Index Array(array=w388, index #1=0 ("index"), index #2=2 ("index")) -> (element #1=w385:string, element #2=w390:string)
    n185 = call "no timeout error.vi"("error in (no error)"=w394) -> ("error out"=w391:errorcluster)
    n186 = Equal?(x="ScanStart", y=w385) -> (x = y?=w382:bool)
    n187 = local read "OK Button"() -> (w393:bool)
    n188 = case shown="True" w382 {
      tunnel: w390 -> [_ w397]
      frame #0 {
      }
      frame #1 {
        "x axis name" <- w397
      }
    }
  }
  n189 = UDP Close(connection ID=w4, 8:w3) -> (error out=→"UDP Mcast Error":errorcluster)  [unwired: 1 out]
